vi "Update Player Who Answered Correctly Last.vi"(8 "error in (no error)":errorcluster, 11 "Controller in":refnum<class "Controller.lvclass">) -> (0 "error out":errorcluster, 3 "Controller out":refnum<class "Controller.lvclass">)   [LabVIEW 2021, in "Controller.lvlib" / "Controller.lvclass"]
uses:
  Controller.lvclass
  Controller.lvclass/Controller.ctl
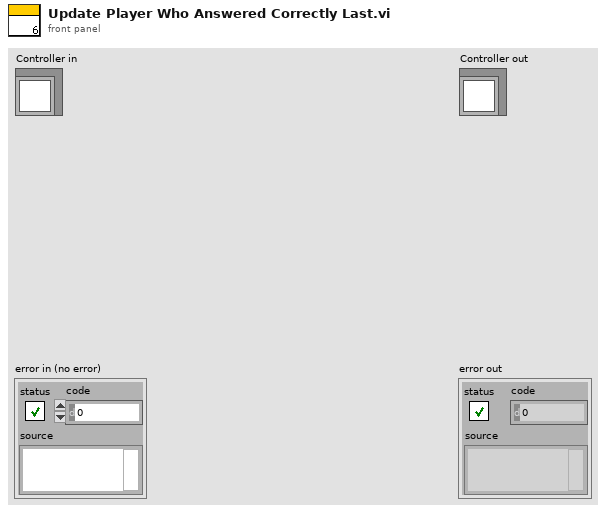
[diagram p1: front panel]
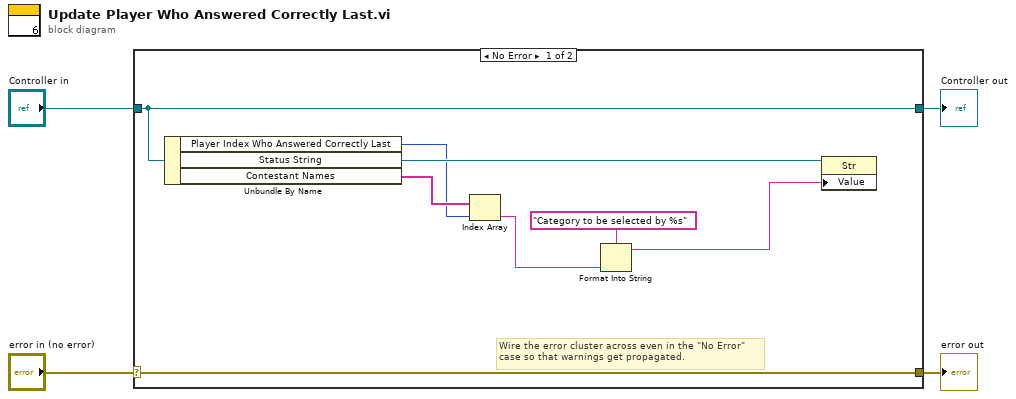
[diagram p0: block diagram]
diagram:
  n1 = case shown="No Error" "error in (no error)" {
    selector: "error in (no error)" -> [w12 w14]
    tunnel: [w12 w14] -> w3
    tunnel: [w6 w13] -> w1
    tunnel: "Controller in" -> [w6 w13]
    frame No Error {
      # "Wire the error cluster across even in the \"No Error\"\ncase so that warnings get propagated."
      n2 = Unbundle By Name(w6) -> ("Player Index Who Answered Correctly Last"=w5:i32, "Status String"=w11:refnum<vi>, "Contestant Names"=w7:string[])
      n3 = Index Array(array=w7, index=w5) -> (element=w9:string)
      n4 = Format Into String(format string="Category to be selected by %s" ("initial string"), w9) -> (resulting string=w8:string)  [unwired: 2 in, 1 out]
      n5 = property class="Str"(reference=w11, "Value"=w8) -> ()  [unwired: 1 in, 2 out]
    }
    frame Error {
    }
  }
  "error out" <- w3
  "Controller out" <- w1
